vi "Main.vi"() -> ()   [LabVIEW 2018]
uses:
  <vilib>/MakerHub/LINX/LMH-LINX.lvlib
  MsgTypedef.ctl
  ProcessDataTypedef.ctl
  <vilib>/MakerHub/LINX/Private/Device/Type Defs/Channels.ctl
  <vilib>/MakerHub/LINX/Private/Device/Type Defs/TCP Config.ctl
  <vilib>/MakerHub/LINX/Private/Device/Device.lvlib
  <vilib>/MakerHub/LINX/Private/Type Defs/Interface.ctl
  <vilib>/MakerHub/LINX/Private/Device/Type Defs/LINX Device Config.ctl
  <vilib>/MakerHub/LINX/Private/Type Defs/Platform.ctl
  <vilib>/MakerHub/LINX/Private/Type Defs/LINX Ref.ctl
  <vilib>/MakerHub/LINX/Public/Utilities/Open Serial.vi
  <vilib>/MakerHub/LINX/Public/Peripherals/Digital/Digital Read 1 Chan.vi
  <vilib>/MakerHub/LINX/Public/Peripherals/Analog/Analog Read 1 Chan.vi
  <vilib>/MakerHub/LINX/Public/Peripherals/Digital/Digital Write 1 Chan.vi
panel:
  out "Target":bool
  in  "TimerON":bool
  in  "TimerCount(ms)":i32=1000
  out "Loop Rate (Hz)":u32
  in  "Close":bool
  in  "Link":bool
  in  "AI Channel":u8
  out "Analog Data":dbl(graph)
  in  "DI Channel":u8=2
  out "DI Value":bool
  in  "DO Value":bool
  in  "DO Channel":u8=3
  in  "Serial Port":refnum<visa-resource-name>
  # "如何把資料送到arduino 上面呢？？"
  # "需求....\n1. linx 連結Arduino board \n2. 即時反應IO狀態\n3. 從VI panel 下達IO控制\n4. 可能作狀態觸發 record 記錄到檔案？\n5. 其它想法...."
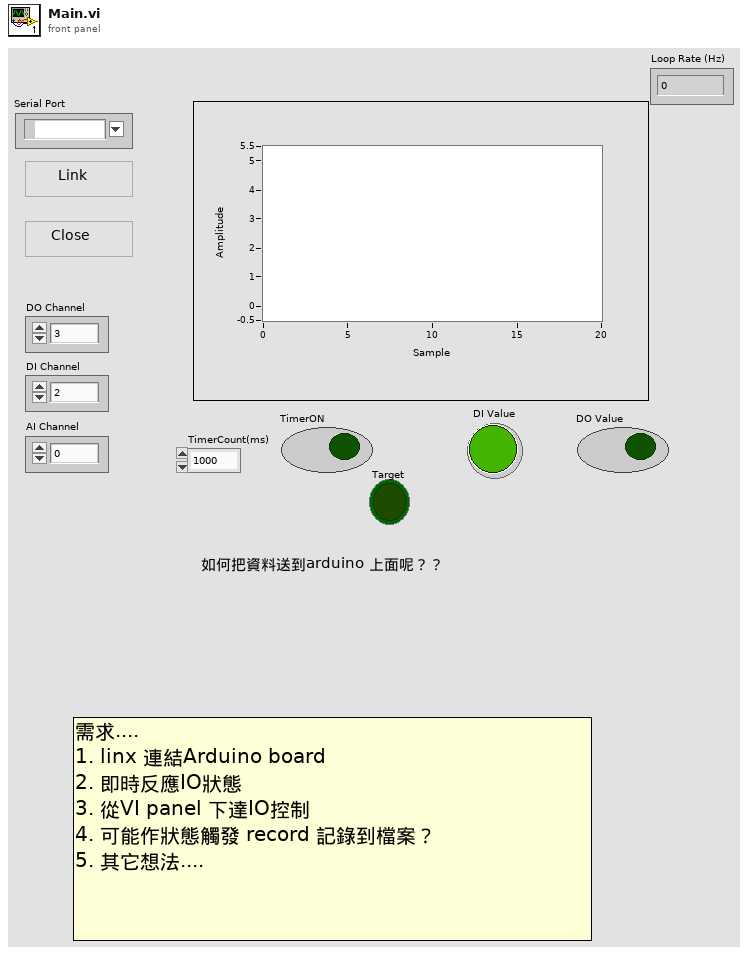
[diagram p1: front panel]
types:
  T1 = typedef "MsgTypedef.ctl" = cluster{"CMD":string, "DATA":variant}
  T2 = typedef "ProcessDataTypedef.ctl" = cluster{"SerialPort":refnum<visa-resource-name>, "DO Channel":u8, "DI Channel":u8, "AI Channel":u8, "AIValue":dbl, "DOStatus":bool, "DIStatus":bool, "DeviceName":string, "LINXResource":T3}
  T3 = typedef "LMH-LINX.lvlib/LINX Ref.ctl" = cluster{"IO":T4, "Interface":T5, "LINX Device Config":T6}
  T4 = typedef "LMH-LINX.lvlib/Platform.ctl" = enum16{"Remote", "Local"}
  T5 = typedef "LMH-LINX.lvlib/Interface.ctl" = enum16{"Serial", "TCP"}
  T6 = typedef "LMH-LINX.lvlib/Device.lvlib/LINX Device Config.ctl" = cluster{"Interface":T5, "COM Port":refnum<visa-resource-name>, "TCP Configuration":T7, "Device Family":u8, "Device ID":u8, "Device Name":string, "TCP Ref":refnum<k5>, "Channels":T8}
  T7 = typedef "LMH-LINX.lvlib/Device.lvlib/TCP Config.ctl" = cluster{"IP Address":string, "Port":u16}
  T8 = typedef "LMH-LINX.lvlib/Channels.ctl" = cluster{"DI":u8[], "DO":u8[], "AI":u8[], "AO":u8[], "PWM":u8[], "QE":u8[], "UART":u8[], "I2C 2":u8[], "SPI":u8[], "CAN":u8[], "Servo":u8[], "AI Ref (V)":dbl, "AI Resolution (Bits)":u8, "AO Ref (V)":dbl, "AO Resolution (Bits)":u8}
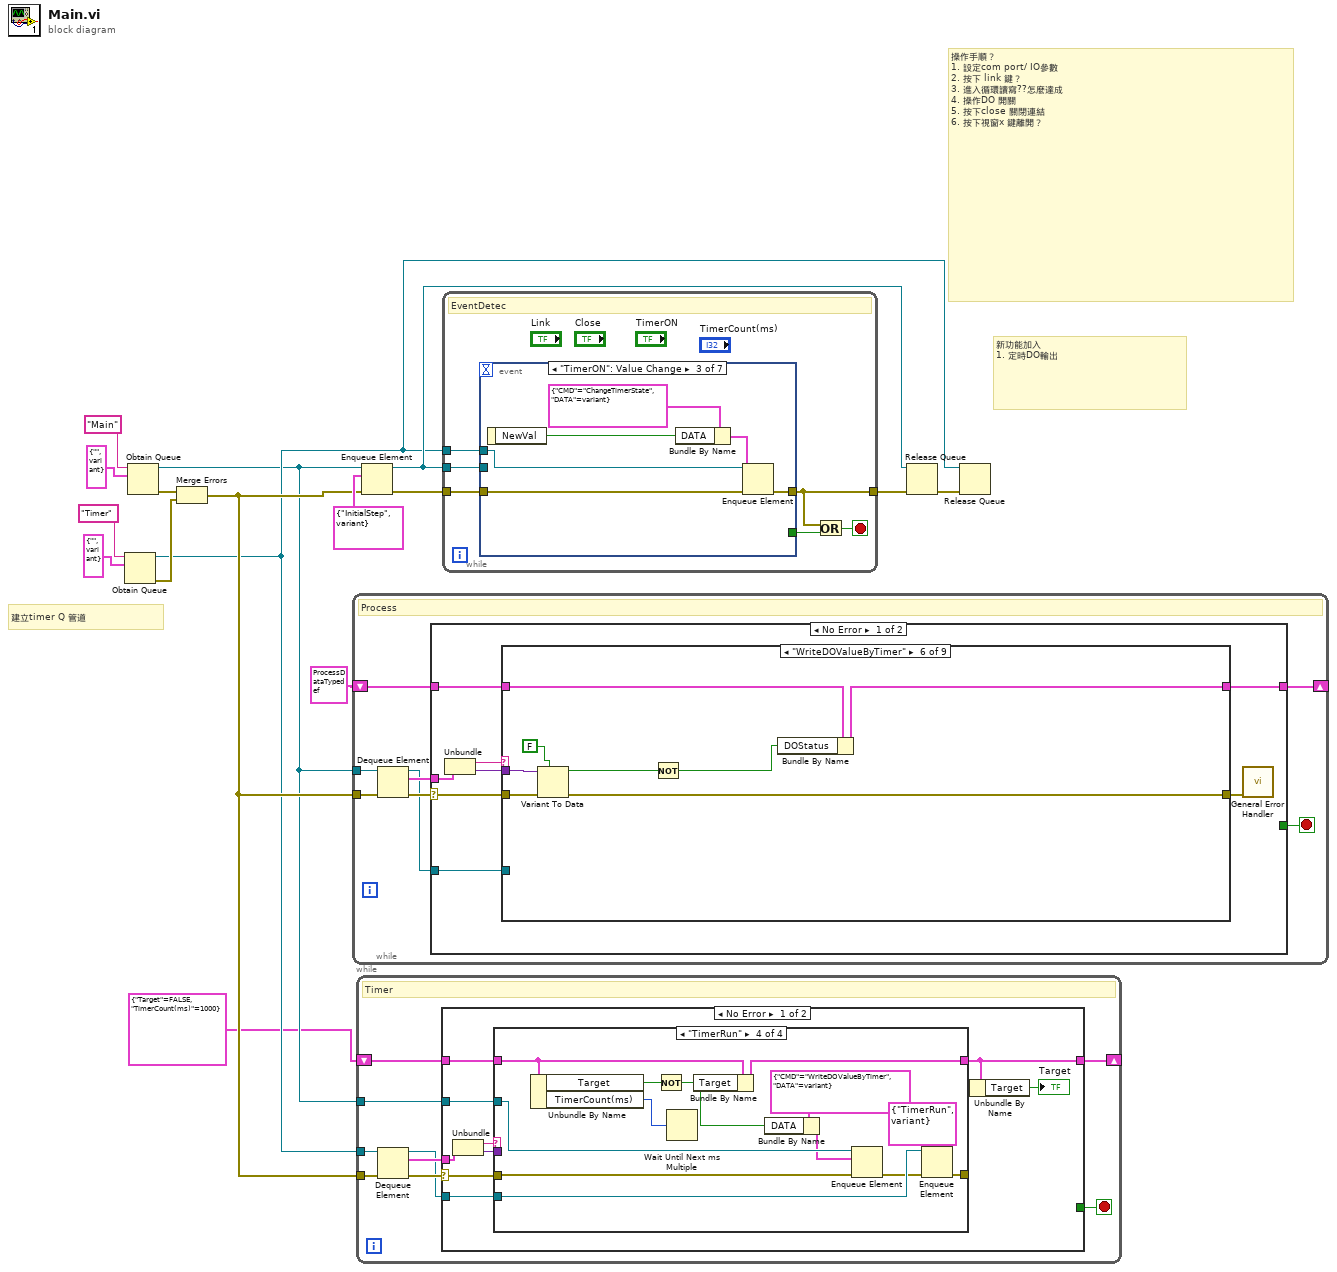
[diagram p0: block diagram]
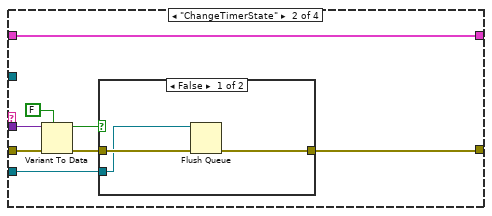
[diagram p3: hidden frame]
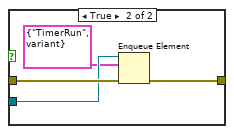
[diagram p4: hidden frame]
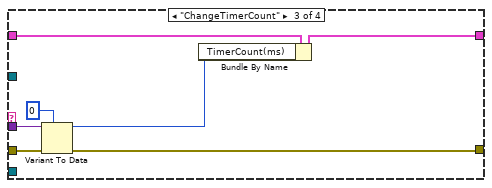
[diagram p5: hidden frame]
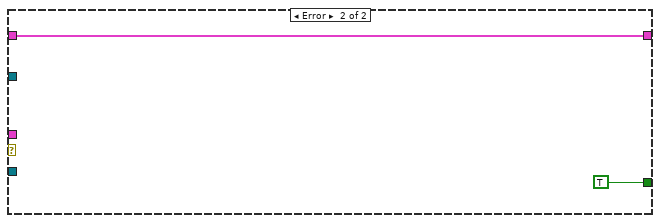
[diagram p6: hidden frame]
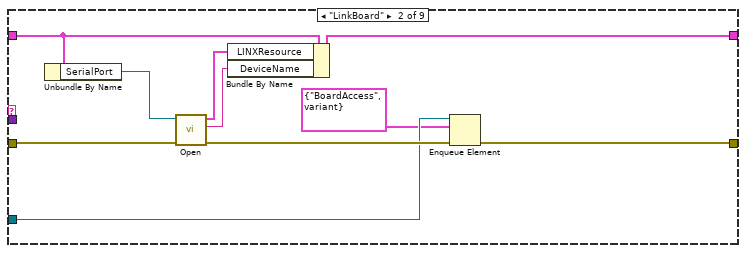
[diagram p8: hidden frame]
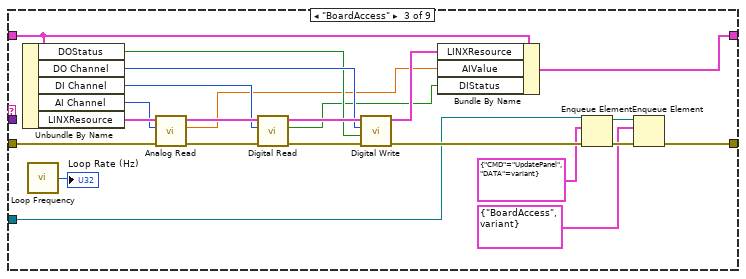
[diagram p9: hidden frame]
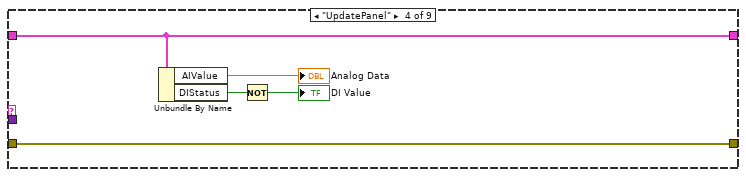
[diagram p10: hidden frame]
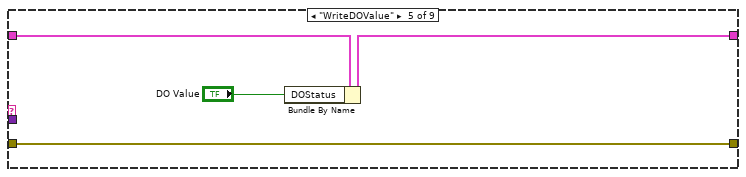
[diagram p11: hidden frame]
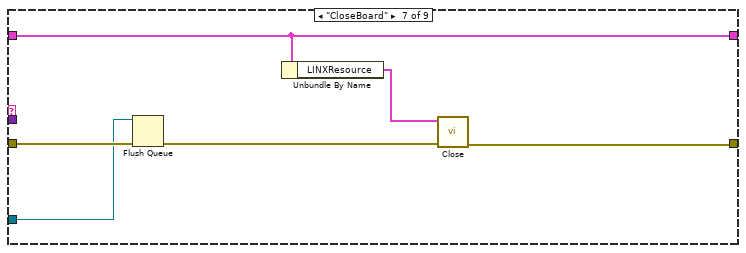
[diagram p12: hidden frame]
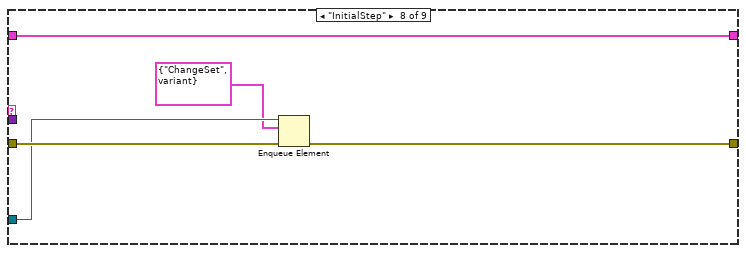
[diagram p13: hidden frame]
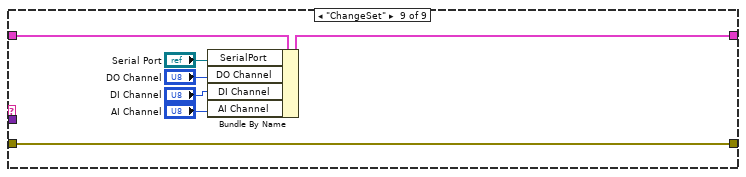
[diagram p14: hidden frame]
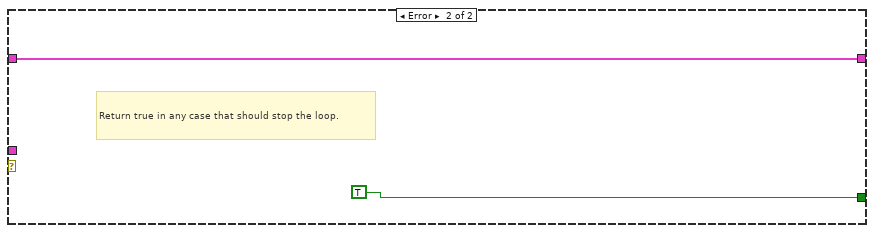
[diagram p15: hidden frame]
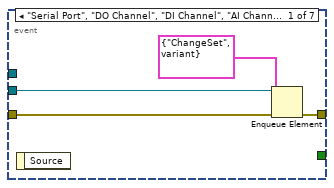
[diagram p16: hidden frame]
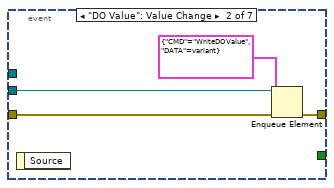
[diagram p17: hidden frame]
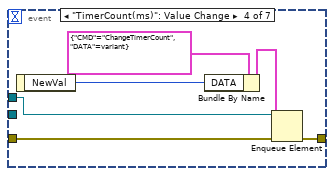
[diagram p18: hidden frame]
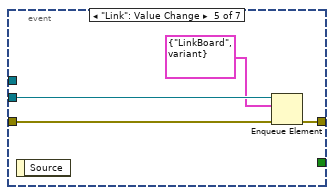
[diagram p19: hidden frame]
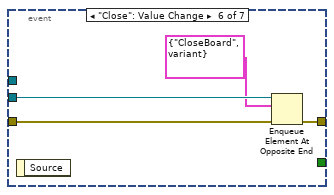
[diagram p20: hidden frame]
diagram:
  # "建立timer Q 管道"
  # "新功能加入\n1. 定時DO輸出"
  # "操作手順？\n1. 設定com port/ IO參數\n2. 按下 link 鍵？\n3. 進入循環讀寫??怎麼達成\n4. 操作DO 開關\n5. 按下close 關閉連結\n6. 按下視窗x 鍵離開？"
  n1 = Obtain Queue(name (unnamed)="Timer", element data type=T1 {"CMD"="", "DATA"=variant}) -> (queue out=w3:refnum<queue>, error out=w6:errorcluster)  [unwired: 3 in, 1 out]
  n2 = Obtain Queue(name (unnamed)="Main", element data type=T1 {"CMD"="", "DATA"=variant}) -> (queue out=w2:refnum<queue>, error out=w16:errorcluster)  [unwired: 3 in, 1 out]
  n3 = Merge Errors(w16, w6) -> (w4:errorcluster)
  n4 = while {
    tunnel: w2 -> [w24]
    shift-right: [w20] -> _
    shift-left: T2 {"SerialPort"="", "DO Channel"=13, "DI Channel"=2, "AI Channel"=0, "AIValue"=0.0, "DOStatus"=FALSE, "DIStatus"=FALSE, "DeviceName"="", "LINXResource"={"IO"=enum."Remote", "Interface"=enum."Serial", "LINX Device Config"={"Interface"=enum."Serial", "COM Port"="COM13", "TCP Configuration"={"IP Address"="", "Port"=0}, "Device Family"=1, "Device ID"=1, "Device Name"="myRIO-1900", "TCP Ref"=refnum, "Channels"={"DI"=[0, 1, 2, 3, 4, 5, 6, 7, 8, 9, 10, 11, 12, 13, 14, 15, 16, 17, 18, 19, 20, 21, 22, 23, 24, 25, 26, 27, 28, 29, 30, 31, 32, 33, 34, 35, 36, 37, 38, 39, 40, 41, 42, 43, 44, 45, 46], "DO"=[0, 1, 2, 3, 4, 5, 6, 7, 8, 9, 10, 11, 12, 13, 14, 15, 16, 17, 18, 19, 20, 21, 22, 23, 24, 25, 26, 27, 28, 29, 30, 31, 32, 33, 34, 35, 36, 37, 38, 39, 40, 41, 42, 43, 44, 45, 46], "AI"=[0, 1, 2, 3, 4, 5, 6, 7, 8, 9, 10, 11], "AO"=[], "PWM"=[3, 5, 6, 9, 10], "QE"=[], "UART"=[0, 1], "I2C 2"=[0], "SPI"=[0], "CAN"=[], "Servo"=[], "AI Ref (V)"=0.0, "AI Resolution (Bits)"=0, "AO Ref (V)"=0.0, "AO Resolution (Bits)"=0}}}} -> [w19]
    tunnel: w4 -> [w17]
    stop <- w21 stop-if-true
    # "Process"
    n5 = Dequeue Element(queue=w24, error in (no error)=w17) -> (queue out=w18:refnum<queue>, element=w22:T1, error out=w23:errorcluster)  [unwired: 1 in, 1 out]
    n6 = case shown="No Error" w23 {
      selector: w23 -> [w30 _]
      tunnel: w22 -> [w32 _]
      tunnel: [_ TRUE] -> w21
      tunnel: [w29 w103] -> w20
      tunnel: w19 -> [w28 w103]
      tunnel: w18 -> [w26 _]
      frame No Error {
        n7 = Unbundle(w32) -> ("CMD"=w31:string, "DATA"=w27:variant)
        n8 = case shown="\"WriteDOValueByTimer\"" w31 {
          tunnel: w30 -> [w33 w44 w62 w72 w75 w83 w90 w94 w96]
          tunnel: [w34 w40 w59 w71 w74 w82 w88 w95 w101] -> w29
          tunnel: w28 -> [w34 w42 w61 w71 w76 w84 w88 w95 w102]
          tunnel: w27 -> [_ _ _ _ _ w80 _ _ _]
          tunnel: [w33 w37 w47 w72 w75 w81 w89 w93 w96] -> w25
          tunnel: w26 -> [_ w36 w49 _ _ _ w85 w92 _]
          frame Default {
          }
          frame "LinkBoard" {
            n9 = Unbundle By Name(w42) -> ("SerialPort"=w41:refnum<visa-resource-name>)
            n10 = call-poly <vilib>:"Open.vi"("Error In"=w44, "Serial Port"=w41) -> ("Error Out"=w43:errorcluster, "Device Name"=w38:string, "LINX Resource"=w39:T3)  [unwired: 7 in]
            n11 = Bundle By Name(cluster=w42, "LINXResource"=w39, "DeviceName"=w38) -> (w40:T2)
            n12 = Enqueue Element(queue=w36, element=T1 {"CMD"="BoardAccess", "DATA"=variant}, error in (no error)=w43) -> (error out=w37:errorcluster)  [unwired: 1 in, 2 out]
          }
          frame "BoardAccess" {
            n13 = Unbundle By Name(w61) -> ("DOStatus"=w54:bool, "DO Channel"=w55:u8, "DI Channel"=w56:u8, "AI Channel"=w57:u8, "LINXResource"=w60:T3)
            n14 = call <vilib>:"Loop Frequency.vi"() -> ("Loop Rate (Hz)"=→"Loop Rate (Hz)":u32)
            n15 = call-poly <vilib>:"Analog Read.vi"("Error In"=w62, "Analog Channel"=w57, "LINX Resource"=w60) -> ("Error Out"=w66:errorcluster, "Voltage"=w53:dbl, "LINX Resource"=w67:T3)  [unwired: 5 in, 1 out]
            n16 = call-poly <vilib>:"Digital Read.vi"("Error In"=w66, "DI Channel"=w56, "LINX Resource"=w67) -> ("Error Out"=w64:errorcluster, "DI Value"=w52:bool, "LINX Resource"=w65:T3)  [unwired: 6 in]
            n17 = call-poly <vilib>:"Digital Write.vi"("Error In"=w64, "Output Value"=w54, "DO Channel"=w55, "LINX Resource"=w65) -> ("Error Out"=w63:errorcluster, "LINX Resource"=w58:T3)  [unwired: 6 in]
            n18 = Bundle By Name(cluster=w61, "LINXResource"=w58, "AIValue"=w53, "DIStatus"=w52) -> (w59:T2)
            n19 = Enqueue Element(queue=w49, element=T1 {"CMD"="UpdatePanel", "DATA"=variant}, error in (no error)=w63) -> (queue out=w46:refnum<queue>, error out=w50:errorcluster)  [unwired: 1 in, 1 out]
            n20 = Enqueue Element(queue=w46, element=T1 {"CMD"="BoardAccess", "DATA"=variant}, error in (no error)=w50) -> (error out=w47:errorcluster)  [unwired: 1 in, 2 out]
          }
          frame "UpdatePanel" {
            n21 = Unbundle By Name(w71) -> ("AIValue"=→"Analog Data":dbl, "DIStatus"=w70:bool)
            n22 = Not(x=w70) -> (.not. x?=→"DI Value":bool)
          }
          frame "WriteDOValue" {
            n23 = Bundle By Name(cluster=w76, "DOStatus"="DO Value") -> (w74:T2)
          }
          frame "WriteDOValueByTimer" {
            n24 = Variant To Data(error in=w83, type=FALSE, Variant=w80) -> (data=w79:bool, error out=w81:errorcluster)
            n25 = Not(x=w79) -> (.not. x?=w77:bool)
            n26 = Bundle By Name(cluster=w84, "DOStatus"=w77) -> (w82:T2)
          }
          frame "CloseBoard" {
            n27 = Flush Queue(queue=w85, error in (no error)=w90) -> (error out=w86:errorcluster)  [unwired: 2 out]
            n28 = Unbundle By Name(w88) -> ("LINXResource"=w87:T3)
            n29 = call <vilib>:"Close.vi"("Error In"=w86, "LINX Resource"=w87) -> ("Error Out"=w89:errorcluster)  [unwired: 9 in]
          }
          frame "InitialStep" {
            n30 = Enqueue Element(queue=w92, element=T1 {"CMD"="ChangeSet", "DATA"=variant}, error in (no error)=w94) -> (error out=w93:errorcluster)  [unwired: 1 in, 2 out]
          }
          frame "ChangeSet" {
            n31 = Bundle By Name(cluster=w102, "SerialPort"="Serial Port", "DO Channel"="DO Channel", "DI Channel"="DI Channel", "AI Channel"="AI Channel") -> (w101:T2)
          }
        }
        n32 = call <vilib>:"General Error Handler.vi"("error in (no error)"=w25) -> ()  [unwired: 10 in, 5 out]
      }
      frame Error {
        # "Return true in any case that should stop the loop."
      }
    }
  }
  n33 = while {
    tunnel: w4 -> [w112]
    tunnel: w3 -> [w111]
    tunnel: w2 -> [w108]
    shift-right: [w106] -> _
    shift-left: cluster{"Target":bool, "TimerCount(ms)":i32} {"Target"=FALSE, "TimerCount(ms)"=1000} -> [w105]
    stop <- w109 stop-if-true
    # "Timer"
    n34 = Dequeue Element(queue=w111, error in (no error)=w112) -> (queue out=w107:refnum<queue>, element=w110:T1, error out=w113:errorcluster)  [unwired: 1 in, 1 out]
    n35 = case shown="No Error" w113 {
      selector: w113 -> [w117 _]
      tunnel: w110 -> [w122 _]
      tunnel: [_ TRUE] -> w109
      tunnel: w108 -> [w120 _]
      tunnel: w107 -> [w119 _]
      tunnel: [w115 w160] -> w106
      tunnel: w105 -> [w116 w160]
      frame No Error {
        n36 = Unbundle(w122) -> ("CMD"=w121:string, "DATA"=w118:variant)
        n37 = case shown="\"TimerRun\"" w121 {
          tunnel: w120 -> [_ _ _ w150]
          tunnel: w119 -> [_ w126 _ w154]
          tunnel: w118 -> [_ w131 w145 _]
          tunnel: w117 -> [w123 w132 w146 w155]
          tunnel: [w124 w129 w142 w157] -> w115
          tunnel: w116 -> [w124 w129 w143 w159]
          tunnel: [w123 w127 w140 w153] -> _
          frame Default {
          }
          frame "ChangeTimerState" {
            n38 = Variant To Data(error in=w132, type=FALSE, Variant=w131) -> (data=w125:bool, error out=w128:errorcluster)
            n39 = case shown="False" w125 {
              tunnel: w128 -> [w135 w139]
              tunnel: [w134 w138] -> w127
              tunnel: w126 -> [w133 w137]
              frame False {
                n40 = Flush Queue(queue=w133, error in (no error)=w135) -> (error out=w134:errorcluster)  [unwired: 2 out]
              }
              frame True {
                n41 = Enqueue Element(queue=w137, element=T1 {"CMD"="TimerRun", "DATA"=variant}, error in (no error)=w139) -> (error out=w138:errorcluster)  [unwired: 1 in, 2 out]
              }
            }
          }
          frame "ChangeTimerCount" {
            n42 = Variant To Data(error in=w146, type=0, Variant=w145) -> (data=w141:i32, error out=w140:errorcluster)
            n43 = Bundle By Name(cluster=w143, "TimerCount(ms)"=w141) -> (w142:cluster{"Target":bool, "TimerCount(ms)":i32})
          }
          frame "TimerRun" {
            n44 = Unbundle By Name(w159) -> ("Target"=w156:bool, "TimerCount(ms)"=w158:i32)
            n45 = Not(x=w156) -> (.not. x?=w147:bool)
            n46 = Wait Until Next ms Multiple(millisecond multiple=w158) -> ()  [unwired: 1 out]
            n47 = Bundle By Name(cluster=w159, "Target"=w147) -> (w157:cluster{"Target":bool, "TimerCount(ms)":i32})
            n48 = Bundle By Name(cluster=T1 {"CMD"="WriteDOValueByTimer", "DATA"=variant} ("element"), "DATA"=w147) -> (w148:T1)
            n49 = Enqueue Element(queue=w150, element=w148, error in (no error)=w155) -> (error out=w151:errorcluster)  [unwired: 1 in, 2 out]
            n50 = Enqueue Element(queue=w154, element=T1 {"CMD"="TimerRun", "DATA"=variant}, error in (no error)=w151) -> (error out=w153:errorcluster)  [unwired: 1 in, 2 out]
          }
        }
        n51 = Unbundle By Name(w115) -> ("Target"=→"Target":bool)
      }
      frame Error {
      }
    }
  }
  n52 = Enqueue Element(queue=w2, element=T1 {"CMD"="InitialStep", "DATA"=variant}, error in (no error)=w4) -> (queue out=w11:refnum<queue>, error out=w12:errorcluster)  [unwired: 1 in, 1 out]
  n53 = while {
    tunnel: w11 -> [w167]
    tunnel: w12 -> [w166]
    tunnel: [w163] -> w15
    tunnel: w3 -> [w162]
    stop <- w164 stop-if-true
    # "EventDetec"
    n54 = event shown="[2] \"TimerON\": Value Change" {
      selector: _ -> [_ _ _ _ _ _ _]
      dyn-events: _ -> [_ _ _ _ _ _ _]
      timeout: _ -> [_ _ _ _ _ _ _]
      tunnel: w167 -> [w171 w175 _ _ w191 w195 _]
      tunnel: w166 -> [w170 w174 w181 w187 w190 w194 w197]
      tunnel: [w169 w173 w180 w186 w189 w193 w197] -> w163
      tunnel: [_ _ _ _ _ _ w196] -> w165
      tunnel: w162 -> [_ _ w178 w184 _ _ _]
      event "Serial Port", "DO Channel", "DI Channel", "AI Channel": Value Change {
        n55 = event-data() -> ()  [unwired: 1 in, 1 out]
        n56 = Enqueue Element(queue=w171, element=T1 {"CMD"="ChangeSet", "DATA"=variant}, error in (no error)=w170) -> (error out=w169:errorcluster)  [unwired: 1 in, 2 out]
      }
      event "DO Value": Value Change {
        n57 = event-data() -> ()  [unwired: 1 in, 1 out]
        n58 = Enqueue Element(queue=w175, element=T1 {"CMD"="WriteDOValue", "DATA"=variant}, error in (no error)=w174) -> (error out=w173:errorcluster)  [unwired: 1 in, 2 out]
      }
      event "TimerON": Value Change {
        n59 = event-data() -> ("NewVal"=w176:bool)  [unwired: 1 in]
        n60 = Bundle By Name(cluster=T1 {"CMD"="ChangeTimerState", "DATA"=variant} ("element"), "DATA"=w176) -> (w177:T1)
        n61 = Enqueue Element(queue=w178, element=w177, error in (no error)=w181) -> (error out=w180:errorcluster)  [unwired: 1 in, 2 out]
      }
      event "TimerCount(ms)": Value Change {
        n62 = event-data() -> ("NewVal"=w182:i32)  [unwired: 1 in]
        n63 = Bundle By Name(cluster=T1 {"CMD"="ChangeTimerCount", "DATA"=variant} ("element"), "DATA"=w182) -> (w183:T1)
        n64 = Enqueue Element(queue=w184, element=w183, error in (no error)=w187) -> (error out=w186:errorcluster)  [unwired: 1 in, 2 out]
      }
      event "Link": Value Change {
        n65 = event-data() -> ()  [unwired: 1 in, 1 out]
        n66 = Enqueue Element(queue=w191, element=T1 {"CMD"="LinkBoard", "DATA"=variant}, error in (no error)=w190) -> (error out=w189:errorcluster)  [unwired: 1 in, 2 out]
      }
      event "Close": Value Change {
        n67 = event-data() -> ()  [unwired: 1 in, 1 out]
        n68 = Enqueue Element At Opposite End(queue=w195, element=T1 {"CMD"="CloseBoard", "DATA"=variant}, error in (no error)=w194) -> (error out=w193:errorcluster)  [unwired: 1 in, 2 out]
      }
      event Panel Close? {
        w196 = TRUE ("Discard?")
        n69 = event-data() -> ()  [unwired: 1 in, 2 out]
        n70 = event-data("Discard?"=w196) -> ()  [unwired: 1 in, 1 out]
      }
    }
    n71 = Or(x=w163, y=w165) -> (x .or. y?=w164:bool)
  }
  n72 = Release Queue(queue=w11, error in (no error)=w15) -> (error out=w5:errorcluster)  [unwired: 1 in, 2 out]
  n73 = Release Queue(queue=w3, error in (no error)=w5) -> ()  [unwired: 1 in, 3 out]
